vi "Rational_Approximation_(iterated_continued_fraction).vi"(8 "max error (1.0e-6)":dbl=1e-06 format="%.2e", 9 "max denominator (max uint32)":u32=4294967295, 10 "max numerator (max int32)":u32=2147483647, 11 "Orig floating point value":dbl=1.0 format="%.12f") -> (0 "error":dbl format="%.2e", 1 "denominator":u32, 2 "numerator":i32, 3 "value of approximation":dbl format="%.8f", 4 "meets error spec?":bool, 5 "# terms":i32)   [LabVIEW 2016]
doc: "Rational Approximation (iterated, continued fraction)\n - produces the smallest (numerator, denominator) ratio that approximates the original floating point value to within the specified maximum error. The algorithm also allows the user to limit the maximum values allowed for the numerator and denominator.\n The method uses a continued fraction representation of the original floating point value. The advantage of this algorithm is its bounded execution time. Preliminary testing shows a slowest case that is ~5x the time of the fastest case.\n\n The original problem for which this function was devised was to create a repeating analog waveform with minimal end-of-buffer distortion. This distortion can arise whenever the waveform frequency cannot divide evenly into an integer number of analog update cycles. In such cases, the transition from the last value in the buffer back to the first value in the buffer is not exactly as desired. This distortion can generally be significantly reduced if a larger buffer can be created which defines multiple cycles of the waveform.\n An example might be an attempt to produce a 6 kHz waveform using a 100 kHz analog update rate. How large a buffer should be created? How many cycles of the waveform will fit in it? To find the answer, run this subvi using 100 / 6 ~= 16.666667 as the 'orig floating point value' input. The 'numerator' output will be the buffer size (50) and the 'denominator' output will be the # of waveform cycles (3). \n Another example (one that inspired this solution) might be an attempt to produce a 600 Hz waveform using an externally generated 15.625 kHz analog update rate, giving a ratio of ~26.0416667. This results in a numerator (buffer size) of 625 and a denominator (# waveform cycles) of 24."
panel:
  out "errors":dbl[](array[numeric]) format="%.2e"
  out "approximations":dbl[](array[numeric]) format="%.6f"
  out "D[]":u32[](array[numeric])
  out "N[]":u32[](array[numeric])
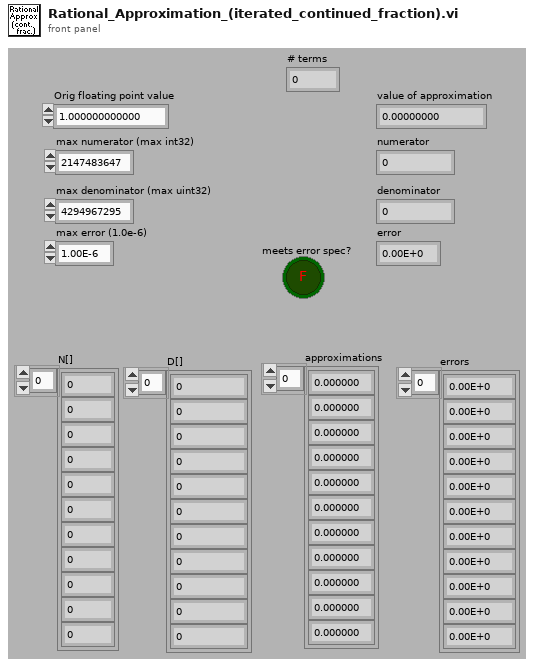
[diagram p1: front panel]
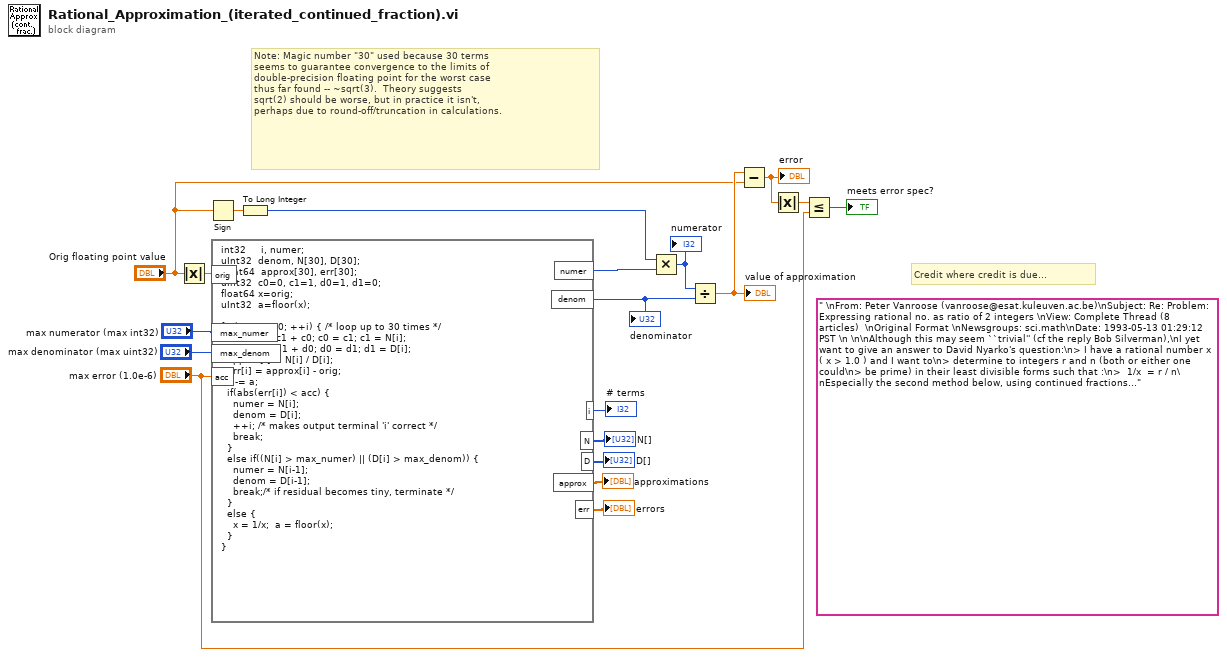
[diagram p0: block diagram]
diagram:
  (unwired) " \nFrom: Peter Vanroose (vanroose@esat.kuleuven.ac.be)\nSubject: Re: Problem: Expressing rational no. as ratio of 2 integers \nView: Complete Thread (8 articles)  \nOriginal Format \nNewsgroups: sci.math\nDate: 1993-05-13 01:29:12 PST \n \n\nAlthough this may seem ``trivial'' (cf the reply Bob Silverman),\nI yet want to give an answer to David Nyarko's question:\n> I have a rational number x ( x > 1.0 ) and I want to\n> determine to integers r and n (both or either one could\n> be prime) in their least divisible forms such that :\n>  1/x  = r / n\nEspecially the second method below, using continued fractions, is interesting.\n\nFirst, it is clear that then x = n / r, still with gcd(n,r)=1.\nSo, let's try to write x as n / r.\n\nFirst method:\nsuppose x is given as 4.6 (short decimal number) or 4 2/16 (fraction)\nor 1/6 + 1/9 (a sum or product of such numbers):\nno problem to immediately write it as 46/10 (fraction with denominator 10^k)\nor 66/16 or 15/54 (put on common denominator, in the last example even\njust straightforward by multiplying denominators).\nThen, simplify by dividing numerator and denominator by their gcd:\n\nint gcd(a, b)\nint a, b; {\n int c;\n if(a < 0) a *= -1;\n if(b < 0) b *= -1;\n if(b < a) c = b, b = a, a = c; /* interchange a and b */\n b %= a;\n return( (b) ? gcd(b,a) : a);\n}\n\n\nSecond method:\nthis will work for `arbitrary' numbers, such as 1.3333333333 (approx. of 4/3)\nor 1.285714 (approx. of 9/7):\nbuild the continued fraction expansion of x by iterating the following:\n- write down the whole part of x (i.e., an integer) and replace x by its\n  fractional part (e.g.: 4.6 -> write down 4 and replace x by 0.6).\n- replace x by 1/x, or stop if x was 0 (or very close to 0).\nreconstruct x from this expansion as follows: e.g., if the expansion is\n(a,b,c,d), then x is\n\n                     1            abcd + ab + ad + cd + 1\n           a + --------------- = -------------------------\n                        1               bcd + b + d\n                b + ---------\n                          1\n                     c + ---\n                          d\nwith nominator and denominator guaranteed to be without common factors.\n\nExample: 1.285714 = [1; 3; 1; 1; 71428; ...] or better (0.000014 ~= 0;\nthe `huge' number 71428 indicates that truncation is recommended):\n         1.285714 ~= [1; 3; 1; 1] = [1; 3; 2], so\n\n                   1            2     9\n           1 + --------- = 1 + --- = ---.\n                     1          7     7\n                3 + ---\n                     2\n\nDetermination of numerator and denominator directly from the continued\nfraction expansion [a0; a1; a2; a3;..an] is possible with the following\nrecursion:\n\nC0 = D1 = 0, C1 = D0 = 1;\nC(m+2) = am * C(m+1) + Cm;\nD(m+2) = am * D(m+1) + Dm.\n\nThe numerator is C(n+2) and the denominator is D(n+2).\n\nExample: 1.285714 ~= [1; 3; 2], thus\nC2 = 1*1+0 = 1, C3 = 3*1+1 = 4, C4 = 2*4+1 = 9.\nD2 = 1*0+1 = 1, D3 = 3*1+0 = 3, D4 = 2*3+1 = 7.\n\nExample: applying this algorithm to 3.14159265 = [3; 7; 15; 1; 288; ...]\ngives   3   22/7   333/106   355/113   102573/32650\nwhere the difference between 355/113 and pi is less than 0.0000003\n(I was told that this approximation of pi was already known in ancient times..)\n\nvoid approx(x, n)\nfloat x;\nint n; {\n int a=x, c0=0, c1=1, d0=1, d1=0, t;\n while(n--) { /* loop n times; infinite loop if n<0 */\n  t = a * c1 + c0; c0 = c1; c1 = t;\n  t = a * d1 + d0; d0 = d1; d1 = t;\n  printf(\"%d/%d\\n\", c1, d1);\n  x -= a;\n  if(x == 0) break;\n  x = 1/x; a = x;\n }\n}\n\nREMARK:\nIt is generally true that the continued fraction approximation Cm / Dm of x\ndiffers from x  by at most 1 / (Dm * D(m+1)) < 1 / square(Dm), i.e.,\nquadratic in the precision.  Moreover, these approximations Cm / Dm are\n``best approximations'' of x, i.e., every rational number which is closer\nto x must have a denominator which is larger than Dm.\n\nREMARK:\nOf course, the continued fraction expansion of x stops iff x is rational.\nBut some irrational numbers have a very regular continued fraction expansion:\n- The expansion *repeats* if and only if x is the root of a second degree\n  polynomial.  E.g., sqrt(2) = [1; 2; 2; 2; 2; ...].\n                     sqrt(3) = [1; 1; 2; 1; 2; ...].\n- The expansion of e ~= 2.71828 is [2; 1; 2; 1; 1; 4; 1; 1; 6; 1; 1; 8; ...]\n\nReference: O. Perron, Die Lehre von den Kettenbr\"uchen, Teubner, 1954.\n\n--\n                                 Peter Vanroose\n                                 Electrotechnical Department, ESAT\n                                 K.U. Leuven, Belgium.\n                                 Peter.Vanroose@esat.kuleuven.ac.be\n\n\n--------------------------------------------------------------------------------\n"
  # "Credit where credit is due..."
  # "Note: Magic number \"30\" used because 30 terms\nseems to guarantee convergence to the limits of \ndouble-precision floating point for the worst case\nthus far found -- ~sqrt(3).  Theory suggests \nsqrt(2) should be worse, but in practice it isn't, \nperhaps due to round-off/truncation in calculations."
  n1 = Absolute Value(x="Orig floating point value") -> (abs(x)=w14:dbl)
  n2 = Sign(1:"Orig floating point value") -> (0:w12:dbl)
  n3 = formula code="int32     i, numer;\nuInt32  denom, N[30], D[30];\nfloat64  approx[30], err[30];\nuInt32  c0=0, c1=1, d0=1, d1=0;\nfloat64 x=orig;\nuInt32  a=floor(x);\n\nfor(i=0; i<30; ++i) { /* loop up to 30 times */\n  N[i] = a * c1 + c0; c0 = c1; c1 = N[i];\n  D[i] = a * d1 + d0; d0 = d1; d1 = D[i];\n  approx[i] = N[i] / D[i];\n  err[i] = approx[i] - orig;\n  x -= a;\n  if(abs(err[i]) < acc) {\n    numer = N[i];\n    denom = D[i];\n    ++i; /* makes output terminal 'i' correct */\n    break;\n  }\n  else if((N[i] > max_numer) || (D[i] > max_denom)) {\n    numer = N[i-1];\n    denom = D[i-1];\n    break;/* if residual becomes tiny, terminate */\n  }\n  else {\n    x = 1/x;  a = floor(x);\n  }\n}"("orig"=w14, "max_numer"="max numerator (max int32)", "max_denom"="max denominator (max uint32)", "acc"="max error (1.0e-6)") -> ("N"=→"N[]":u32[], "D"=→"D[]":u32[], "approx"=→"approximations":dbl[], "i"=→"# terms":i32, "numer"=w10:i32, "denom"=w15:u32, "err"=→"errors":dbl[])
  "denominator" <- w15
  n4 = To Long Integer(number=w12) -> (32bit integer=w11:i32)
  n5 = Multiply(x=w11, y=w10) -> (x*y=w9:i32)
  "numerator" <- w9
  n6 = Divide(x=w9, y=w15) -> (x/y=w8:dbl)
  "value of approximation" <- w8
  n7 = Subtract(x=w8, y="Orig floating point value") -> (x-y=w7:dbl)
  "error" <- w7
  n8 = Absolute Value(x=w7) -> (abs(x)=w6:dbl)
  n9 = Less Or Equal?(x=w6, y="max error (1.0e-6)") -> (x <= y?=→"meets error spec?":bool)
